vi "Prepare header content.vi"(8 "error in (no error)":errorcluster, 11 "Save Image in":refnum<class "Save Image.lvclass">) -> (0 "error out":errorcluster, 2 "cluster of jsons 2":T1, 3 "Save Image out":refnum<class "Save Image.lvclass">)   [LabVIEW 2018, in "Save Image.lvclass"]
doc: "Prepare the header content to be provided to the Python toolkit\n\nThis function returns a JSON with the information to be written into the image header"
uses:
  Save Image.lvclass
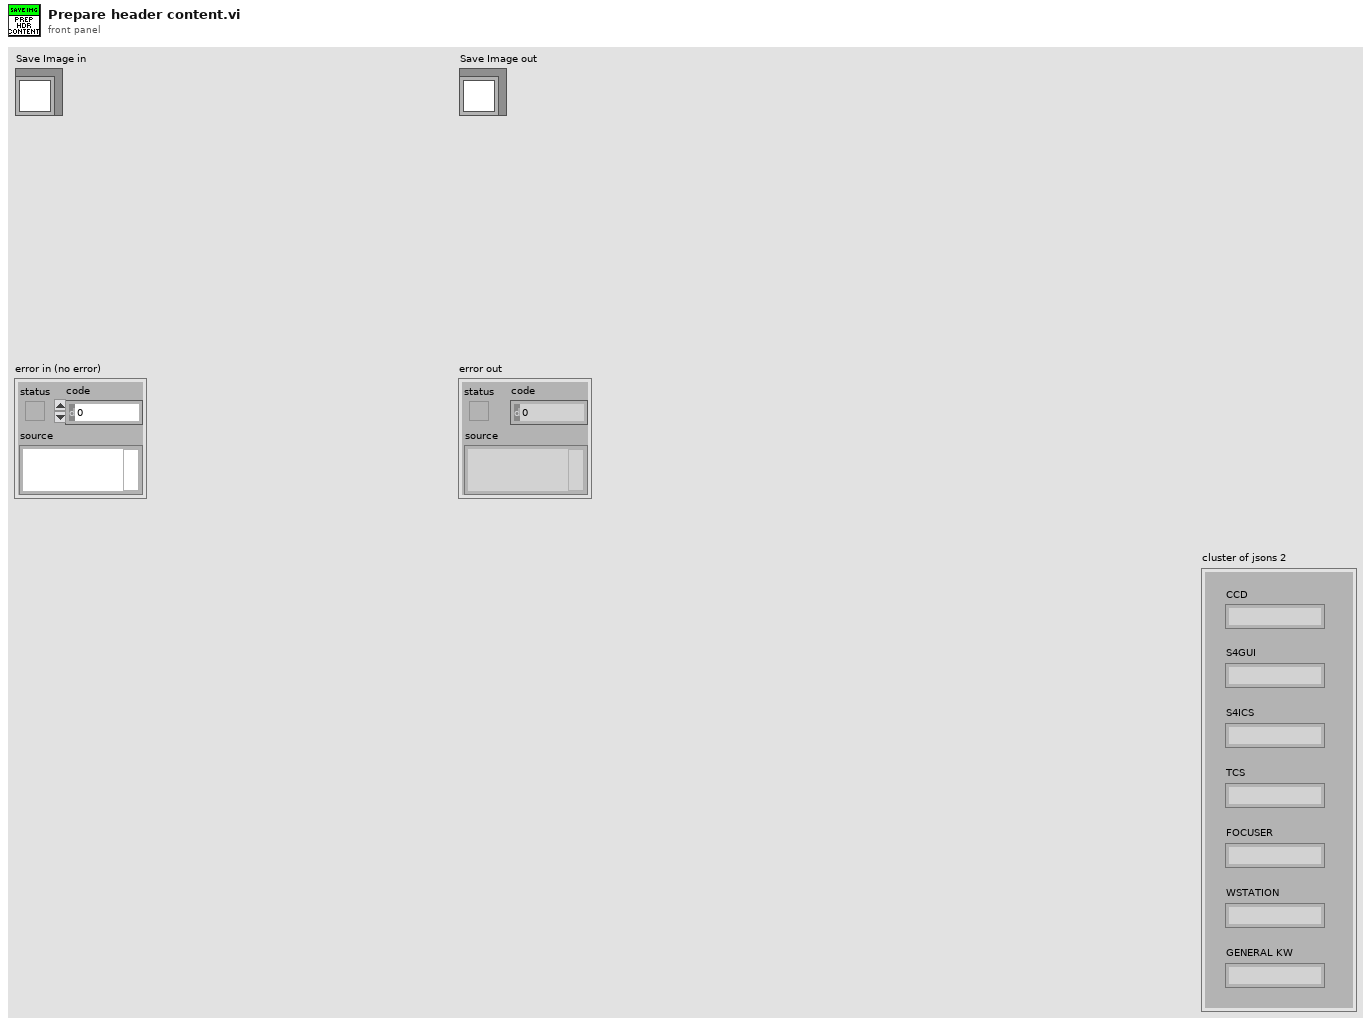
[diagram p1: front panel]
types:
  T1 = cluster{"CCD":string, "S4GUI":string, "S4ICS":string, "TCS":string, "FOCUSER":string, "WSTATION":string, "GENERAL KW":string}
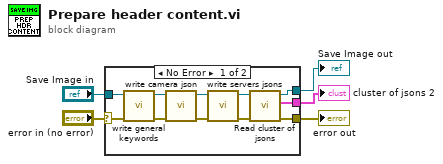
[diagram p0: block diagram]
diagram:
  n1 = case shown="No Error" "error in (no error)" {
    selector: "error in (no error)" -> [w13 w18]
    tunnel: [w8 w18] -> w4
    tunnel: [w9 w17] -> w2
    tunnel: "Save Image in" -> [w14 w17]
    tunnel: [w6 _] -> w1
    frame No Error {
      n2 = call "write general keywords.vi"("error in (no error)"=w13, "Save Image in"=w14) -> ("error out"=w16:errorcluster, "Save Image out"=w15:refnum<class "Save Image.lvclass">)  [unwired: 8 in]
      n3 = call "write camera json.vi"("error in (no error)"=w16, "Save Image in"=w15) -> ("error out"=w11:errorcluster, "Save Image out"=w12:refnum<class "Save Image.lvclass">)  [unwired: 8 in]
      n4 = call "write servers jsons.vi"("error in (no error)"=w11, "Save Image in"=w12) -> ("error out"=w7:errorcluster, "Save Image out"=w10:refnum<class "Save Image.lvclass">)  [unwired: 8 in]
      n5 = call-dynamic "Read cluster of jsons.vi"("error in (no error)"=w7, "Save Image in"=w10) -> ("error out"=w8:errorcluster, "cluster of jsons"=w6:T1, "Save Image out"=w9:refnum<class "Save Image.lvclass">)  [unwired: 7 in]
    }
    frame Error {
    }
  }
  "error out" <- w4
  "Save Image out" <- w2
  "cluster of jsons 2" <- w1
